vi "SubVI_Definindo_ROI_esteira_alterado.vi"(6 "largura_y":sgl=30.0, 7 "largura_x":sgl=30.0, 8 "error in (no error)":errorcluster, 9 "ofset y":sgl, 10 "Session in":T3, 11 "ofset x":sgl) -> (0 "error out":errorcluster, 1 "ROI Descriptor":T4 {"Contours"."Type" items=["No Selection", "Point", "Line", "Rectangle", "Oval", "Polygon", "Freehand Region", "Annulus", "Unused2", "Unused3", "Broken Line", "Freehand Line", "Rotated Rectangle"]}, 3 "Session Out":T3)   [LabVIEW 2017]
uses:
  <vilib>/userdefined/High Color/IMAQdx.ctl
  <vilib>/vision/driver/IMAQdx.llb/IMAQdx Buffer Number Mode.ctl
  <vilib>/vision/NI_Vision_Development_Module.lvlib
  <resource>/objmgr/IMAQImage.rc
  <vilib>/vision/driver/NI_Vision_Acquisition_Software.lvlib
panel:
  out "Matches (pixel)":T1(array[cluster]) {"Bounding Box"."y" format="%.2f"; "Bounding Box"."x" format="%.2f"; "Score" format="%.2f"; "Scale" format="%.2f"; "Angle" format="%.2f"; "Position"."y" format="%.2f"; "Position"."x" format="%.2f"}
  out "Image Out":T2(plugin-control)
  out "error out 2":errorcluster
  out "Imagem Original":T2(plugin-control)
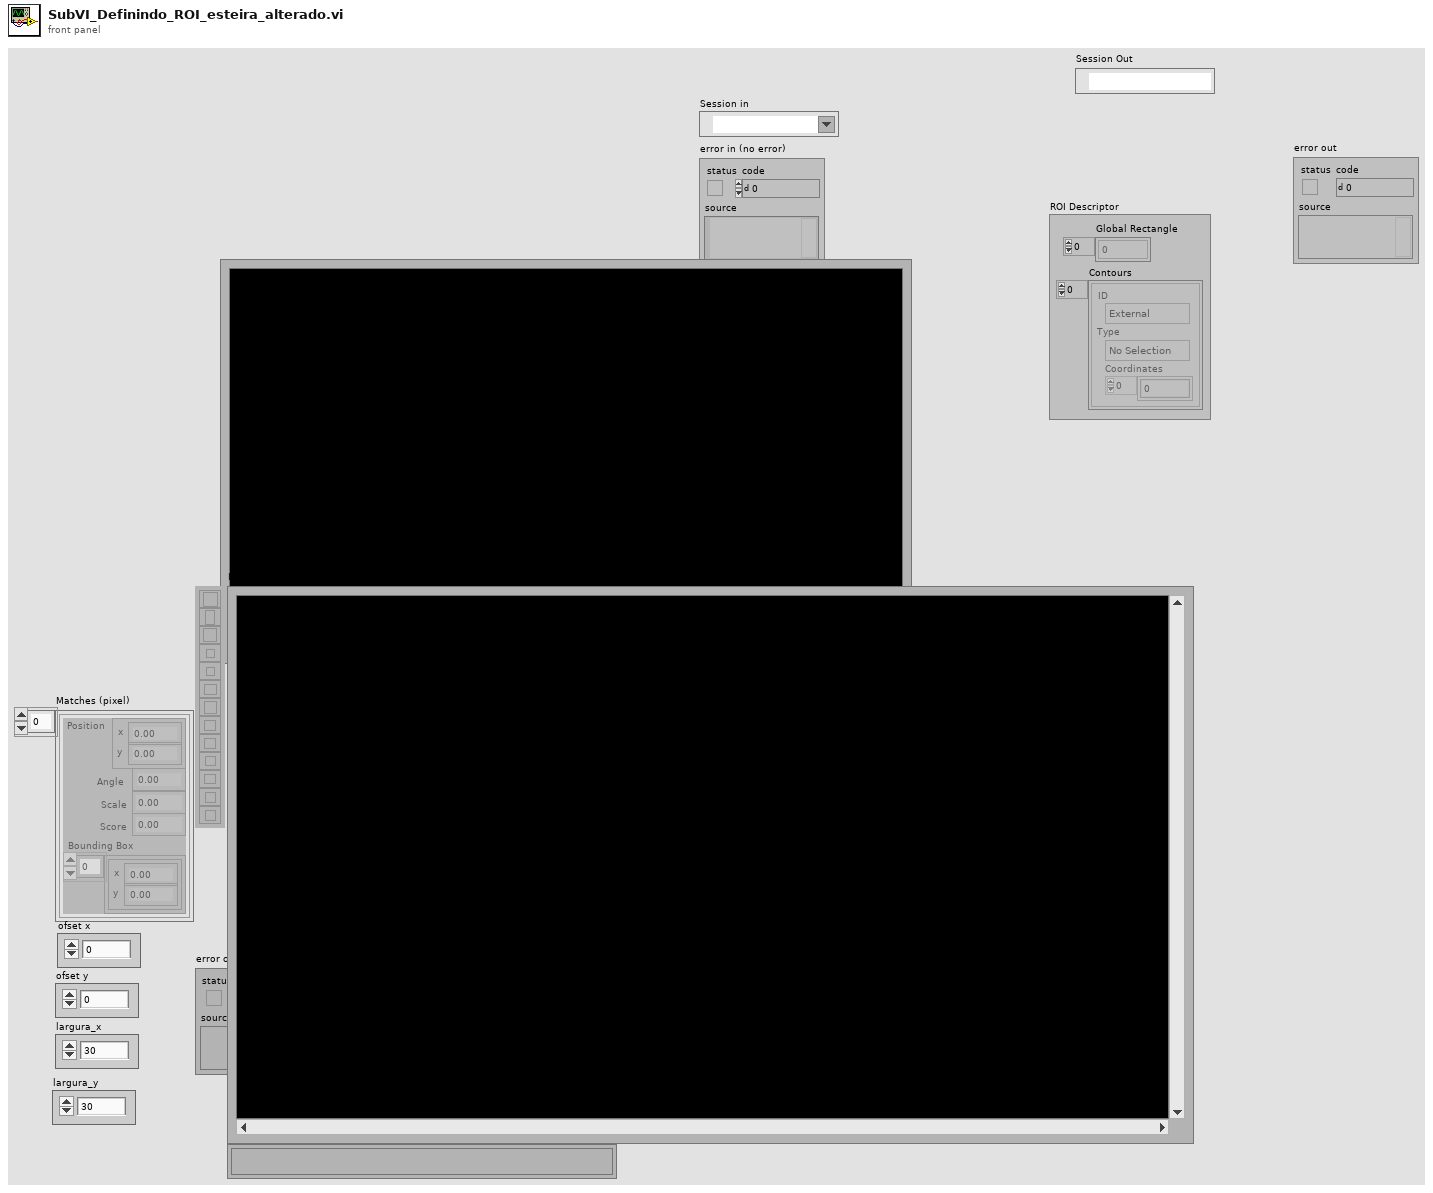
[diagram p1: front panel]
types:
  T1 = cluster{"Position":cluster{"x":sgl, "y":sgl}, "Angle":sgl, "Scale":sgl, "Score":sgl, "Bounding Box":cluster{"x":sgl, "y":sgl}[]}[]
  T2 = typedef "IMAQ Image.ctl" = refnum<image>
  T3 = typedef "IMAQdx.ctl" = refnum<k21>
  T4 = typedef "ROI Descriptor" = cluster{"Global Rectangle":i32[], "Contours":cluster{"ID":enum32{"External", "Internal"}, "Type":u32, "Coordinates":i32[]}[]}
  T5 = cluster{"Number of Matches Requested":i32, "Minimum Match Score":sgl, "Angle Ranges":cluster{"Start Angle":sgl, "End Angle":sgl}[]}
  T6 = cluster{"Global Rectangle":i32[], "Contours":cluster{"ID":enum32{"External", "Internal"}, "Type":u32, "Coordinates":i32[]}[]}
  T7 = typedef "NI_Vision_Acquisition_Software.lvlib/IMAQdx Buffer Number Mode.ctl" = enum32{"Next", "Last", "Buffer Number", "Every", "Last New"}
  T8 = cluster{"histogram":u32[], "Minimal Value":sgl, "Maximal Value":sgl, "Starting Value":sgl, "Interval Width":sgl, "Mean Value":sgl, "Standard  Variation":sgl, "Area (pixels)":i32}
  T9 = typedef "Image Type" = u32
  T10 = cluster{"element":dbl, "y":i32, "x":i32, "element":dbl, "element":dbl}
  T11 = cluster{"Position":cluster{"x":sgl, "y":sgl}, "Angle":sgl, "Scale":sgl, "Score":sgl, "Bounding Box":cluster{"x":sgl, "y":sgl}[]}
  T12 = cluster{"element":dbl, sgl, "x":i32, sgl, "element":dbl}
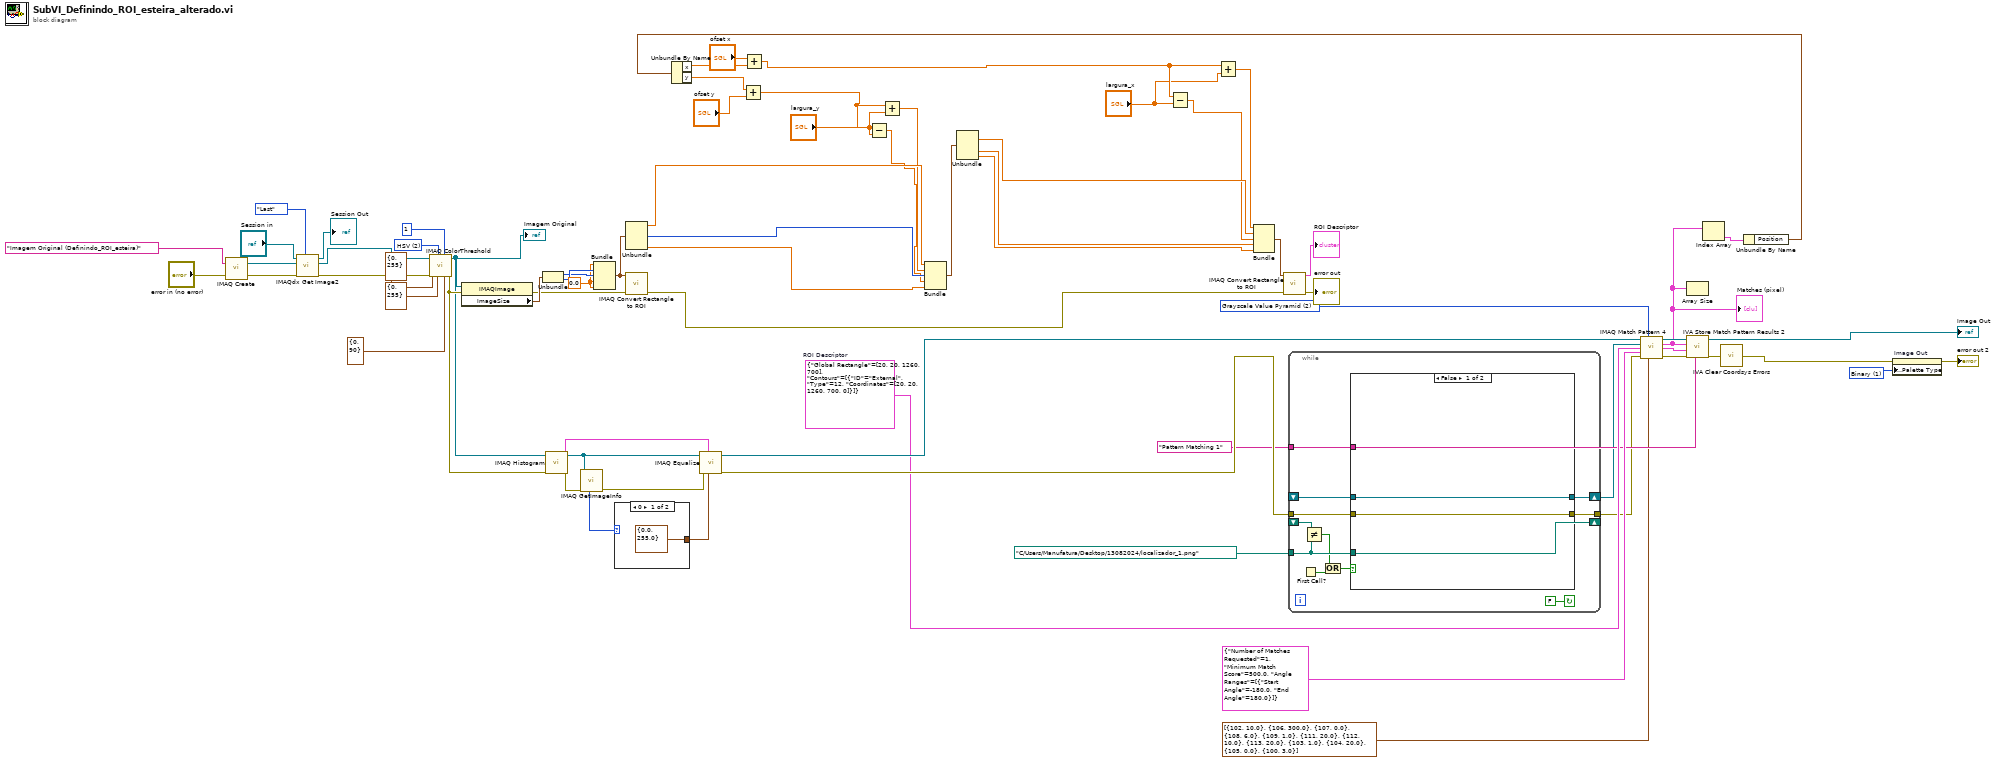
[diagram p0: block diagram]
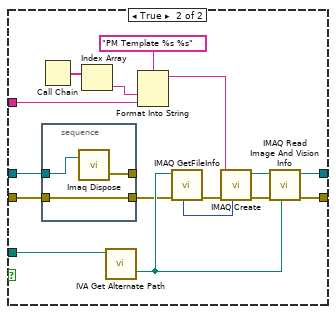
[diagram p2: hidden frame]
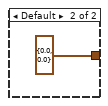
[diagram p3: hidden frame]
diagram:
  w19 = u32 1 items=["Grayscale", "Binary", "Gradient", "Rainbow", "Temperature", "User Defined", "Binary 16 Bit", "Gradient 16 Bit", "Rainbow 16 Bit", "Temperature 16 Bit", "User Defined 16 Bit"] ("Palette Type")
  w31 = 2 items=["All", "Low Discrepancy Sampling", "Grayscale Value Pyramid", "Gradients Pyramid"] ("Algorithm")
  w28 = "Pattern Matching 1" ("Step Name")
  w30 = T6 {"Global Rectangle"=[20, 20, 1260, 700], "Contours"=[{"ID"=enum."External", "Type"=12, "Coordinates"=[20, 20, 1260, 700, 0]}]}  # ROI Descriptor
  w56 = u16 2 items=["RGB", "HSL", "HSV", "HSI"] ("Color Mode")
  w59 = 0.0 ("element")
  n1 = call "IMAQ Create"("Image Name"="Imagem Original (Definindo_ROI_esteira)", "error in (no error)"="error in (no error)") -> ("New Image"=w53:T2, "error out"=w44:errorcluster)  [unwired: 3 in]
  n2 = call <vilib>:"IMAQdx Get Image2.vi"("Buffer Number Mode (Next)"=IMAQdx_Buffer_Number_Mode."Last", "error in"=w44, "Image In"=w53, "Session In"="Session in") -> ("error out"=w42:errorcluster, "Image Out"=w43:T2, "Session Out"=→"Session Out":T3)  [unwired: 4 in, 1 out]
  n3 = call "IMAQ ColorThreshold"("Blue or Luma or Val or Inten Range"=cluster{"Lower value":i32, "Upper value":i32} {"Lower value"=0, "Upper value"=90}, "Replace Value"=1, "Green or Sat Range"=cluster{"Lower value":i32, "Upper value":i32} {"Lower value"=0, "Upper value"=255}, "Color Mode"=w56, "error in (no error)"=w42, "Red or Hue Range"=cluster{"Lower value":i32, "Upper value":i32} {"Lower value"=0, "Upper value"=255}, "Image Src"=w43) -> ("error out"=w18:errorcluster, "Image Dst Out"=w2:T2)  [unwired: 1 in, 2 out]
  "Imagem Original" <- w2
  n4 = property class="IMAQImage"(reference=w2, error in=w18) -> (error out=w50:errorcluster, "ImageSize"=w58:cluster{"x":i32, "y":i32})  [unwired: 1 out]
  n5 = Unbundle(w58) -> ("x"=w60:i32, "y"=w61:i32)
  n6 = call "IMAQ Histogram"("error in (no error)"=w18, "Image"=w2) -> ("error out"=w38:errorcluster, "Histogram Report"=w40:T8)  [unwired: 3 in, 5 out]
  n7 = call "IMAQ GetImageInfo"("error in (no error)"=w38, "Image"=w2) -> ("error out"=w37:errorcluster, "Image Type"=w39:T9)  [unwired: 8 out]
  n8 = Bundle("element"=w59, "y"=w61, "x"=w60, "element"=w59, "element"=w59) -> (w66:T10)  [unwired: 1 in]
  n9 = case shown="0" w39 {
    tunnel: [cluster{"Minimum":sgl, "Maximum":sgl} {"Minimum"=0.0, "Maximum"=255.0} ("Range") cluster{"Minimum":sgl, "Maximum":sgl} {"Minimum"=0.0, "Maximum"=0.0} ("Range")] -> w36
    frame 0 {
    }
    frame Default {
    }
  }
  n10 = Unbundle(w66) -> ("element"=w63:dbl, "x"=w62:i32, "element"=w64:dbl)  [unwired: 2 out]
  n11 = call "IMAQ Convert Rectangle to ROI"("error in (no error)"=w50, "Rectangle"=w66) -> ("error out"=w1:errorcluster)  [unwired: 7 in, 1 out]
  n12 = call "IMAQ Equalize"("Range"=w36, "Histogram Report"=w40, "error in (no error)"=w37, "Image Src"=w2) -> ("error out"=w41:errorcluster, "Image Dst Out"=w34:T2)  [unwired: 2 in, 4 out]
  n13 = while {
    shift-right: [w84] -> w26
    shift-left: _ -> [w83]
    tunnel: [w81] -> w25
    tunnel: w41 -> [w80]
    tunnel: path "C:/Users/Manufatura/Desktop/13082024/localizador_1.png" ("Template File Path") -> [w77]
    tunnel: w28 -> [w79]
    shift-right: [w77] -> _
    shift-left: _ -> [w78]
    stop <- FALSE continue-if-true
    n14 = First Call?() -> (First Call?: T/F=w76:bool)
    n15 = Not Equal?(x=w78, y=w77) -> (x != y?=w75:bool)
    n16 = Or(x=w75, y=w76) -> (x .or. y?=w74:bool)
    n17 = case shown="False" w74 {
      tunnel: [w86 w100] -> w84
      tunnel: w83 -> [w86 w92]
      tunnel: [w85 w97] -> w81
      tunnel: w80 -> [w85 w91]
      tunnel: w77 -> [_ w93]
      tunnel: w79 -> [_ w94]
      frame False {
      }
      frame True {
        n18 = stacked-sequence {
          tunnel: w92 -> [w105]
          tunnel: w91 -> [w104]
          tunnel: [w104] -> w87
          tunnel: [w103] -> _
          frame #0 {
            n19 = call "Imaq Dispose"("Image"=w105) -> ("error out"=w103:errorcluster)  [unwired: 2 in, 3 out]
          }
        }
        n20 = Call Chain() -> (call chain=w96:string[])
        n21 = Index Array(array=w96) -> (element=w95:string)  [unwired: 1 in]
        n22 = call <vilib>:"IVA Get Alternate Path.vi"("Path In"=w93) -> ("Path Out"=w89:path)  [unwired: 10 out]
        n23 = Format Into String(format string="PM Template %s %s" ("Image Name"), w95, w94) -> (resulting string=w102:string)  [unwired: 2 in, 1 out]
        n24 = call "IMAQ GetFileInfo"("error in (no error)"=w87, "File Path"=w89) -> ("error out"=w88:errorcluster, "Image Type"=w90:T9)  [unwired: 3 in, 5 out]
        n25 = call "IMAQ Create"("Image Name"=w102, "Image Type"=w90, "error in (no error)"=w88) -> ("New Image"=w99:T2, "error out"=w98:errorcluster)  [unwired: 1 in, 1 out]
        n26 = call "IMAQ Read Image And Vision Info"("File Path"=w89, "error in (no error)"=w98, "Image"=w99) -> ("error out"=w97:errorcluster, "Image Out"=w100:T2)  [unwired: 1 in, 6 out]
      }
    }
  }
  n27 = call "IMAQ Match Pattern 4"("Image"=w34, "Algorithm"=w31, "Template Image"=w26, "ROI Descriptor"=w30, "Parameters"=T5 {"Number of Matches Requested"=1, "Minimum Match Score"=500.0, "Angle Ranges"=[{"Start Angle"=-180.0, "End Angle"=180.0}]}, "error in (no error)"=w25, "Advanced Options"=cluster{"Item":u16, "Value":dbl}[] [{"Item"=102, "Value"=10.0}, {"Item"=106, "Value"=300.0}, {"Item"=107, "Value"=0.0}, {"Item"=108, "Value"=6.0}, {"Item"=109, "Value"=1.0}, {"Item"=111, "Value"=20.0}, {"Item"=112, "Value"=10.0}, {"Item"=113, "Value"=20.0}, {"Item"=103, "Value"=1.0}, {"Item"=104, "Value"=20.0}, {"Item"=105, "Value"=0.0}, {"Item"=100, "Value"=3.0}]) -> ("Image (duplicate)"=w32:T2, "Matches (pixel)"=w17:T1, "Matches (real-world)"=w27:T1, "error out"=w33:errorcluster)  [unwired: 4 in, 1 out]
  "Matches (pixel)" <- w17
  n28 = Array Size(array=w17) -> ()  [unwired: 1 out]
  n29 = call <vilib>:"IVA Store Match Pattern Results 2.vi"("Step Name"=w28, "error in (no error)"=w33, "Matches (real-world)"=w27, "Matches (pixel)"=w17, "Image in"=w32) -> ("error out"=w24:errorcluster, "Image dup"=→"Image Out":T2)  [unwired: 1 in, 4 out]
  n30 = Index Array(array=w17) -> (element=w16:T11)  [unwired: 1 in]
  n31 = call <vilib>:"IVA Clear Coordsys Errors.vi"("error in (no error)"=w24) -> ("error out"=w23:errorcluster)  [unwired: 10 in]
  n32 = Unbundle By Name(w16) -> ("Position"=w15:cluster{"x":sgl, "y":sgl})
  n33 = Unbundle By Name(w15) -> ("x"=w9:sgl, "y"=w6:sgl)
  n34 = Add(x=w6, y="ofset y") -> (x+y=w7:sgl)
  n35 = Add(x="ofset x", y=w9) -> (x+y=w10:sgl)
  n36 = Subtract(x=w7, y="largura_y") -> (x-y=w13:sgl)
  n37 = Add(x=w7, y="largura_y") -> (x+y=w14:sgl)
  n38 = Bundle("element"=w63, w14, "x"=w62, w13, "element"=w64) -> (w68:T12)  [unwired: 1 in]
  n39 = Unbundle(w68) -> (w69:sgl, w70:sgl, "element"=w67:dbl)  [unwired: 2 out]
  n40 = Subtract(x=w10, y="largura_x") -> (x-y=w11:sgl)
  n41 = Add(x=w10, y="largura_x") -> (x+y=w12:sgl)
  n42 = Bundle(w12, w69, w11, w70, "element"=w67) -> (w65:cluster{sgl, sgl, sgl, sgl, "element":dbl})  [unwired: 1 in]
  n43 = call "IMAQ Convert Rectangle to ROI"("error in (no error)"=w1, "Rectangle"=w65) -> ("error out"=→"error out":errorcluster, "ROI Descriptor"=→"ROI Descriptor":T4)  [unwired: 7 in]
  n44 = property on="Image Out" class="ImageControl"(error in=w23, "Palette:Palette Type"=w19) -> (error out=→"error out 2":errorcluster)  [unwired: 1 in, 1 out]
